vi "zapis.vi"(0 "Byte Stream File Refnum":refnum<file>, 5 "error in (no error)":errorcluster, 6 "Ciecz in":T1={"Thin [C]"=20.0, "V"=0.0025, "cw [J/(kg*K)]"=4200.0, "ro [kg/m3]"=997.0, "F1 [m2]"=2.0, "Ph"=11400.0, "Pnom"=20.0, "h"=1.0}, 7 "Zapis do pliku":bool, 8 "thout":dbl, 10 "probka":dbl) -> (14 "Byte Stream File Refnum 2":refnum<file>, 19 "error out":errorcluster)   [LabVIEW 2023]
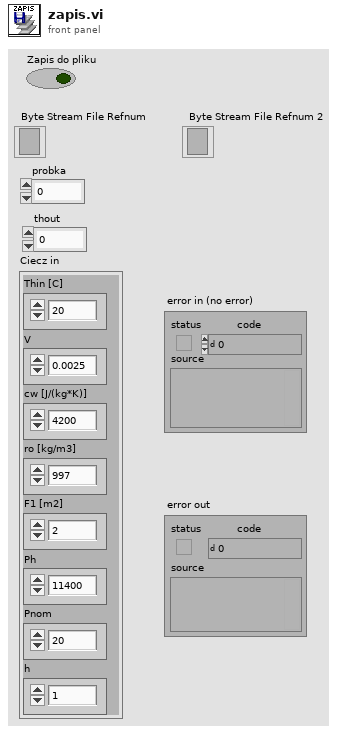
[diagram p1: front panel]
types:
  T1 = cluster{"Thin [C]":dbl, "V":dbl, "cw [J/(kg*K)]":dbl, "ro [kg/m3]":dbl, "F1 [m2]":dbl, "Ph":dbl, "Pnom":dbl, "h":dbl}
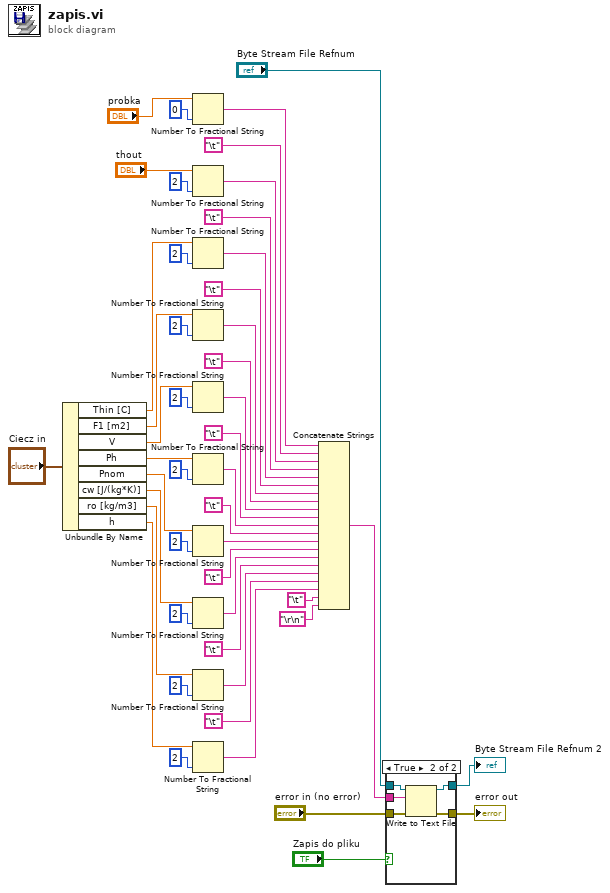
[diagram p0: block diagram]
diagram:
  n1 = Unbundle By Name("Ciecz in") -> ("Thin [C]"=w31:dbl, "F1 [m2]"=w30:dbl, "V"=w29:dbl, "Ph"=w28:dbl, "Pnom"=w27:dbl, "cw [J/(kg*K)]"=w26:dbl, "ro [kg/m3]"=w25:dbl, "h"=w24:dbl)
  n2 = Number To Fractional String(number="probka", precision (6)=i16 0) -> (F-format string=w40:string)  [unwired: 2 in]
  n3 = Number To Fractional String(number="thout", precision (6)=i16 2) -> (F-format string=w43:string)  [unwired: 2 in]
  n4 = Number To Fractional String(number=w31, precision (6)=i16 2) -> (F-format string=w45:string)  [unwired: 2 in]
  n5 = Number To Fractional String(number=w30, precision (6)=i16 2) -> (F-format string=w47:string)  [unwired: 2 in]
  n6 = Number To Fractional String(number=w29, precision (6)=i16 2) -> (F-format string=w23:string)  [unwired: 2 in]
  n7 = Number To Fractional String(number=w28, precision (6)=i16 2) -> (F-format string=w21:string)  [unwired: 2 in]
  n8 = Number To Fractional String(number=w27, precision (6)=i16 2) -> (F-format string=w19:string)  [unwired: 2 in]
  n9 = Number To Fractional String(number=w26, precision (6)=i16 2) -> (F-format string=w17:string)  [unwired: 2 in]
  n10 = Number To Fractional String(number=w25, precision (6)=i16 2) -> (F-format string=w15:string)  [unwired: 2 in]
  n11 = Number To Fractional String(number=w24, precision (6)=i16 2) -> (F-format string=w13:string)  [unwired: 2 in]
  n12 = Concatenate Strings(w40, "\t", w43, "\t", w45, "\t", w47, "\t", w23, "\t", w21, "\t", w19, "\t", w17, "\t", w15, "\t", w13, "\t", "\r\n") -> (w38:string)
  n13 = case shown="True" "Zapis do pliku" {
    tunnel: w38 -> [_ w55]
    tunnel: "Byte Stream File Refnum" -> [w49 w54]
    tunnel: "error in (no error)" -> [w50 w53]
    tunnel: [w50 w52] -> w34
    tunnel: [w49 w51] -> w33
    frame False {
    }
    frame True {
      n14 = Write to Text File(file (use dialog)=w54, text=w55, error in=w53) -> (refnum out=w51:refnum<file>, error out=w52:errorcluster)  [unwired: 1 in, 1 out]
    }
  }
  "error out" <- w34
  "Byte Stream File Refnum 2" <- w33
